vi "CRYGet Tree Number by StepNo.vi"(10 "sOption":string, 11 "Step Setup VI No":i32) -> (2 "Number in SubSequence":string, 3 "Number in Tree":i32)   [LabVIEW 2013]
uses:
  CRYProject Editor Global.vi
  CRYCurveLibrary/Global/CRYCurve Library Global.vi
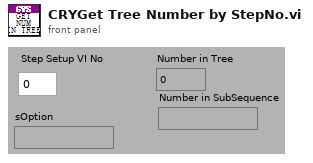
[diagram p1: front panel]
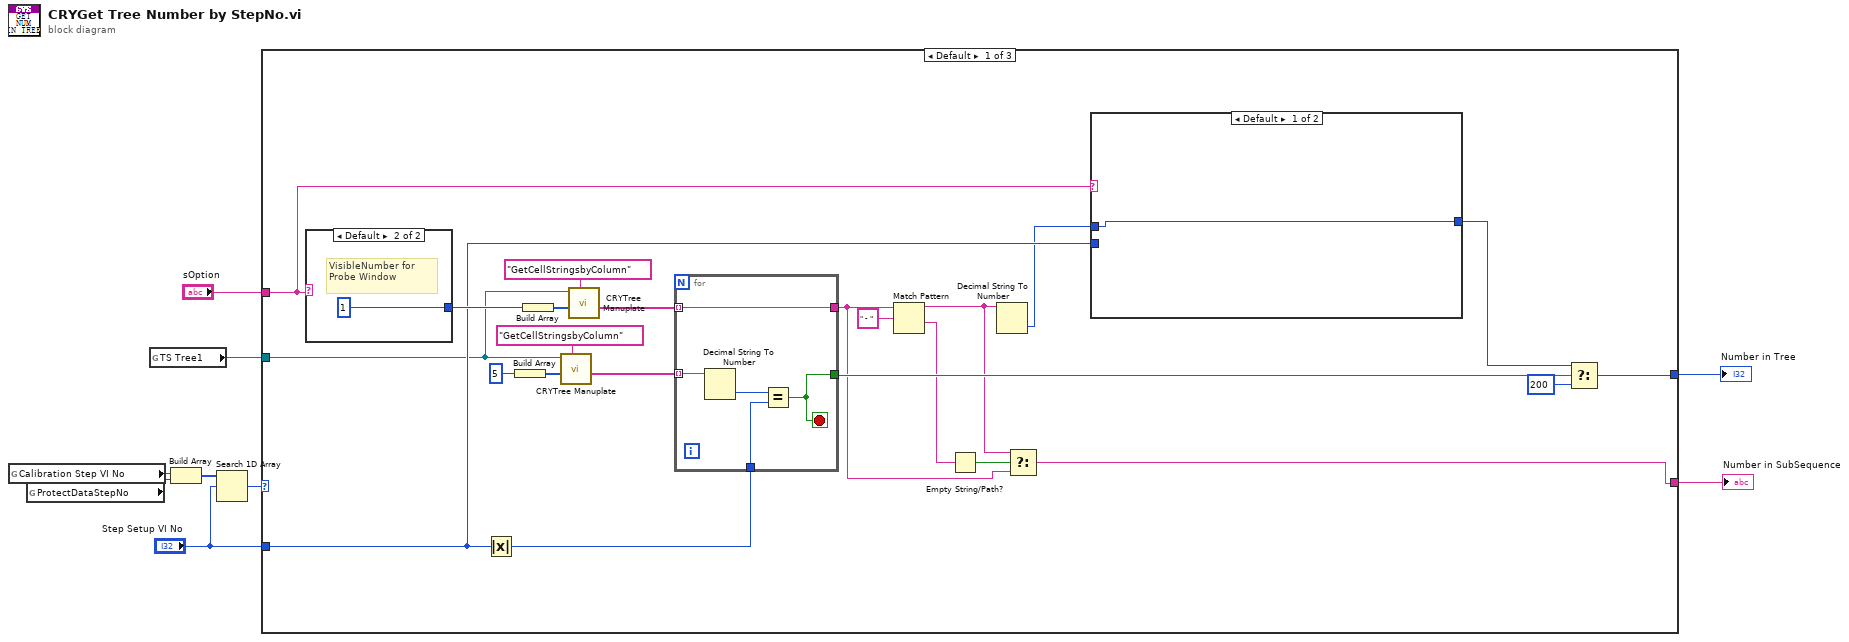
[diagram p0: block diagram]
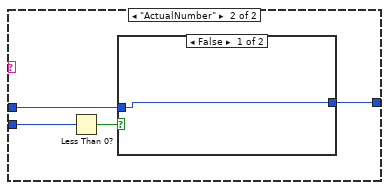
[diagram p2: hidden frame]
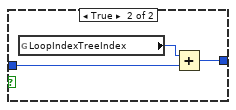
[diagram p3: hidden frame]
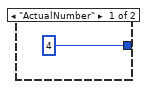
[diagram p4: hidden frame]
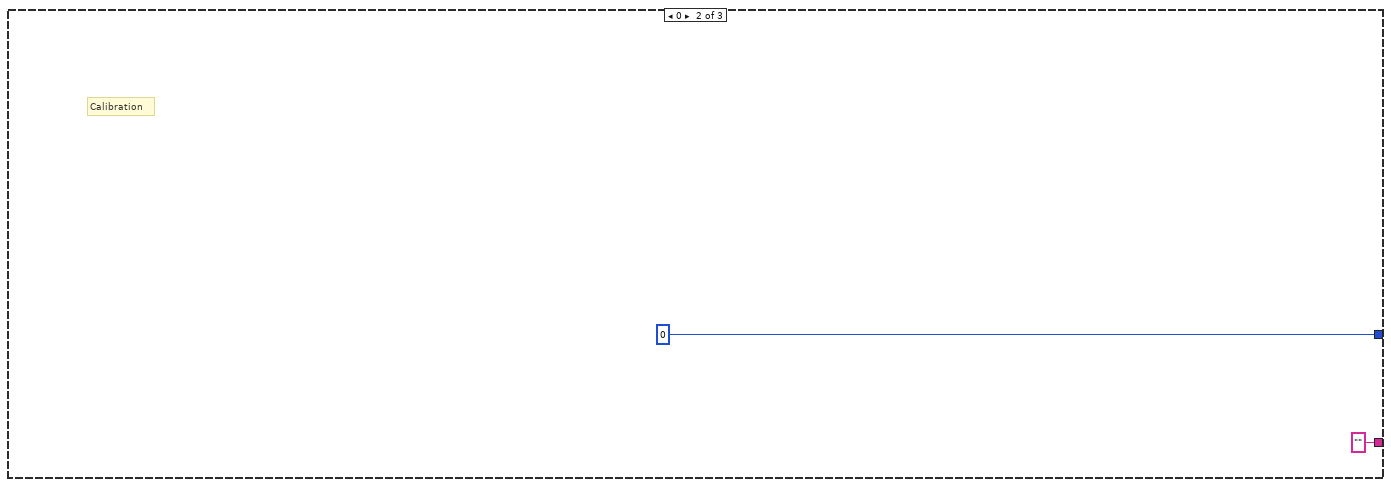
[diagram p5: hidden frame]
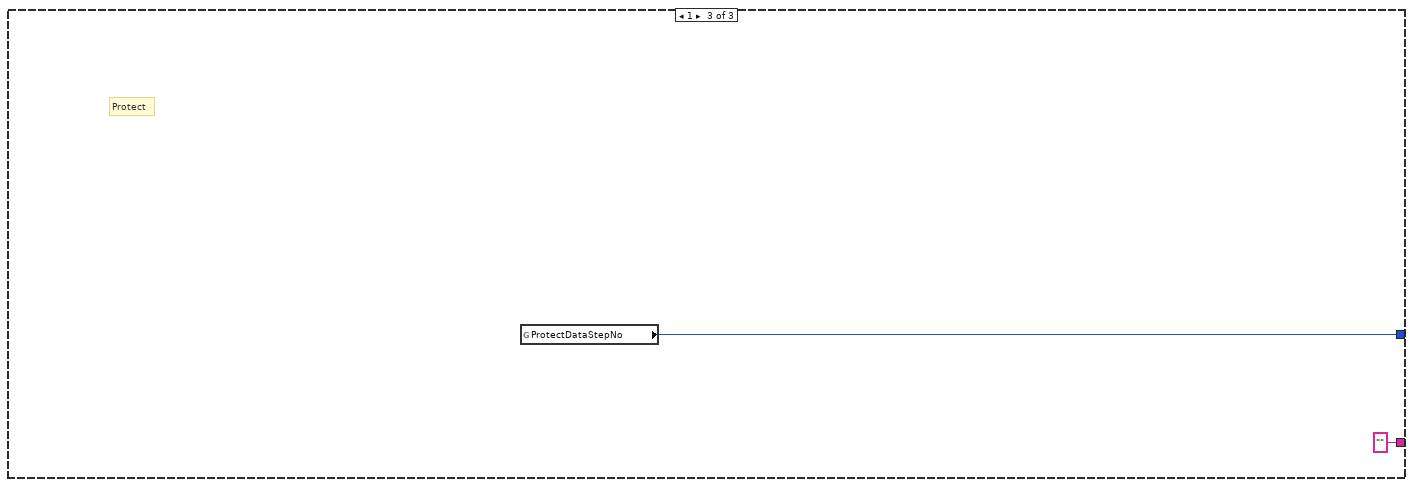
[diagram p6: hidden frame]
diagram:
  n1 = global read "CRYProject Editor Global.vi" "Calibration Step VI No"() -> (w5:i32)
  n2 = global read "CRYCurve Library Global.vi" "ProtectDataStepNo"() -> (w4:i32)
  n3 = global read "CRYProject Editor Global.vi" "TS Tree1"() -> (w8:refnum<vi>)
  n4 = Build Array(w5, w4) -> (w3:i32[])
  n5 = Search 1D Array(1D array=w3, element="Step Setup VI No") -> (index of element=w1:i32)  [unwired: 1 in]
  n6 = case shown="Default" w1 {
    tunnel: [w22 0 ("f") w52] -> w9
    tunnel: "Step Setup VI No" -> [w20 _ _]
    tunnel: w8 -> [w18 _ _]
    tunnel: [w10 "" ("Navigate Tree:Get Child") "" ("Navigate Tree:Get Child")] -> w7
    tunnel: "sOption" -> [w17 _ _]
    frame Default {
      n7 = case shown="Default" w17 {
        tunnel: [4 ("nData 2") 1 ("nData 2")] -> w27
        frame "ActualNumber" {
        }
        frame Default {
          # "VisibleNumber for\nProbe Window"
        }
      }
      n8 = Absolute Value(x=w20) -> (abs(x)=w24:i32)
      n9 = Build Array(5 ("nData 2")) -> (w30:i32[])
      n10 = Build Array(w27) -> (w28:i32[])
      n11 = call "CRYTree Manuplate.vi"("sAction"="GetCellStringsbyColumn", "nData"=w30, "Tree in"=w18) -> ("sData Out"=w29:string[])  [unwired: 5 in, 3 out]
      n12 = call "CRYTree Manuplate.vi"("sAction"="GetCellStringsbyColumn", "nData"=w28, "Tree in"=w18) -> ("sData Out"=w25:string[])  [unwired: 5 in, 3 out]
      n13 = for {
        tunnel: w29 -> [w48] mode=indexing
        tunnel: w24 -> [w47]
        tunnel: w25 -> [w46] mode=indexing
        tunnel: [w46] -> w11
        tunnel: [w44] -> w23
        stop <- w44 stop-if-true
        n14 = Decimal String To Number(string=w48) -> (number=w45:i32)  [unwired: 2 in, 1 out]
        n15 = Equal?(x=w45, y=w47) -> (x = y?=w44:bool)
      }
      n16 = Match Pattern(string=w11, regular expression=" - " ("format string")) -> (before substring=w12:string, after substring=w14:string)  [unwired: 1 in, 2 out]
      n17 = Empty String/Path?(string/path=w14) -> (empty?=w13:bool)
      n18 = Decimal String To Number(string=w12) -> (number=w16:i32)  [unwired: 2 in, 1 out]
      n19 = Select(t=w12, s=w13, f=w11) -> (s? t:f=w10:string)
      n20 = case shown="Default" w17 {
        tunnel: w20 -> [_ w36]
        tunnel: w16 -> [w33 w35]
        tunnel: [w33 w34] -> w19
        frame Default {
        }
        frame "ActualNumber" {
          n21 = Less Than 0?(x=w36) -> (x < 0?=w37:bool)
          n22 = case shown="False" w37 {
            tunnel: w35 -> [w38 w41]
            tunnel: [w38 w39] -> w34
            frame False {
            }
            frame True {
              n23 = global read "CRYCurve Library Global.vi" "LoopIndexTreeIndex"() -> (w40:i32)
              n24 = Add(x=w40, y=w41) -> (x+y=w39:i32)
            }
          }
        }
      }
      n25 = Select(t=w19, s=w23, f=200) -> (s? t:f=w22:i32)
    }
    frame 0 {
      # "Calibration"
    }
    frame 1 {
      # "Protect"
      n26 = global read "CRYCurve Library Global.vi" "ProtectDataStepNo"() -> (w52:i32)
    }
  }
  "Number in Tree" <- w9
  "Number in SubSequence" <- w7
